vi "EnvironmentStepAnanlysisModule.vi"(0 "AnalysisContext":refnum<k7>) -> (1 "status":bool, 2 "code":i32, 3 "source":string)   [LabVIEW 2013]
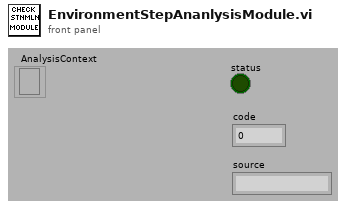
[diagram p1: front panel]
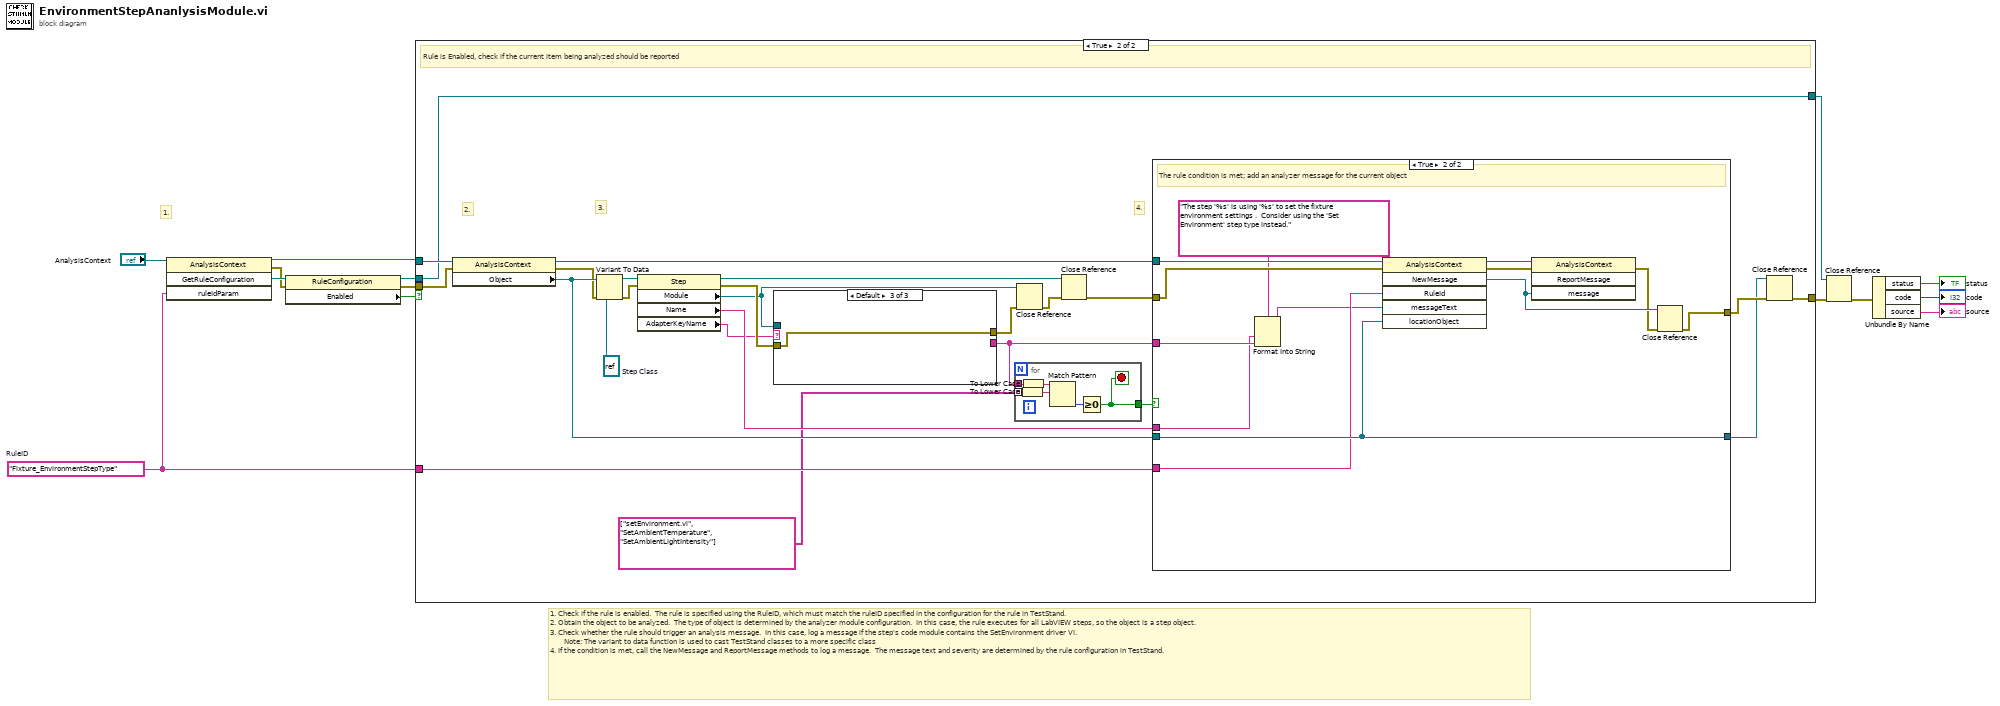
[diagram p0: block diagram]
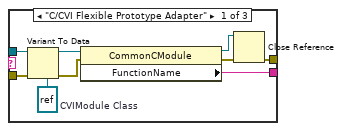
[diagram p3: hidden frame]
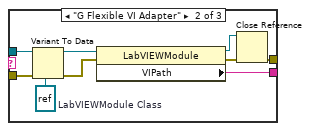
[diagram p4: hidden frame]
diagram:
  w6 = "Fixture_EnvironmentStepType"  # RuleID
  # "1. Check if the rule is enabled.  The rule is specified using the RuleID, which must match the ruleID specified in the configuration for the rule in TestStand.\n2. Obtain the object to be analyzed.  The type of object is determined by the analyzer module configuration.  In this case, the rule executes for all LabVIEW steps, so the object is a step object.\n3. Check whether the rule should trigger an analysis message.  In this case, log a message if the step's code module contains the SetEnvironment driver VI.  \n       Note: The variant to data function is used to cast TestStand classes to a more specific class\n4. If the condition is met, call the NewMessage and ReportMessage methods to log a message.  The message text and severity are determined by the rule configuration in TestStand."
  # "1."
  n1 = invoke class="AnalysisContext" method="GetRuleConfiguration"(reference="AnalysisContext", "ruleIdParam"=w6) -> (reference out=w10:refnum<k7>, error out=w12:errorcluster, "GetRuleConfiguration"=w13:refnum<k7>)  [unwired: 2 in, 1 out]
  n2 = property class="RuleConfiguration"(reference=w13, error in=w12) -> (reference out=w5:refnum<k7>, error out=w4:errorcluster, "Enabled"=w11:bool)
  n3 = case shown="True" w11 {
    tunnel: w4 -> [w16 w19]
    tunnel: [w16 w27] -> w3
    tunnel: w10 -> [_ w23]
    tunnel: w6 -> [_ w25]
    tunnel: w5 -> [w15 w20]
    tunnel: [w15 w20] -> w2
    frame False {
      # "Rule is Disabled, do nothing"
    }
    frame True {
      w39 = refnum<k7> refnum  # Step Class
      # "4."
      # "3."
      # "2."
      # "Rule is Enabled, check if the current item being analyzed should be reported"
      n4 = property class="AnalysisContext"(reference=w23, error in=w19) -> (reference out=w40:refnum<k7>, error out=w18:errorcluster, "Object"=w29:refnum<k7>)
      n5 = Variant To Data(error in=w18, type=w39, Variant=w29) -> (data=w38:refnum<k7>, error out=w37:errorcluster)
      n6 = property class="Step"(reference=w38, error in=w37) -> (reference out=w31:refnum<k7>, error out=w36:errorcluster, "Module"=w33:refnum<k7>, "Name"=w24:string, "AdapterKeyName"=w17:string)
      n7 = case shown="Default" w17 {
        tunnel: w36 -> [w47 w62 w65]
        tunnel: [w49 w58 w65] -> w34
        tunnel: w33 -> [w52 w57 _]
        tunnel: [w50 w56 _] -> w22
        frame "C/CVI Flexible Prototype Adapter" {
          w51 = refnum<k7> refnum  # CVIModule Class
          n8 = Variant To Data(error in=w47, type=w51, Variant=w52) -> (data=w55:refnum<k7>, error out=w54:errorcluster)
          n9 = property class="CommonCModule"(reference=w55, error in=w54) -> (reference out=w48:refnum<k7>, error out=w53:errorcluster, "FunctionName"=w50:string)
          n10 = Close Reference(reference=w48, error in (no error)=w53) -> (error out=w49:errorcluster)
        }
        frame "G Flexible VI Adapter" {
          w64 = refnum<k7> refnum  # LabVIEWModule Class
          n11 = Variant To Data(error in=w62, type=w64, Variant=w57) -> (data=w63:refnum<k7>, error out=w61:errorcluster)
          n12 = property class="LabVIEWModule"(reference=w63, error in=w61) -> (reference out=w60:refnum<k7>, error out=w59:errorcluster, "VIPath"=w56:string)
          n13 = Close Reference(reference=w60, error in (no error)=w59) -> (error out=w58:errorcluster)
        }
        frame Default {
        }
      }
      n14 = for {
        tunnel: [w41] -> w35
        tunnel: w22 -> [w43]
        tunnel: string[] ["setEnvironment.vi", "SetAmbientTemperature", "SetAmbientLightIntensity"] -> [w42] mode=indexing
        stop <- w41 stop-if-true
        n15 = To Lower Case(string=w42) -> (all lower case string=w45:string)
        n16 = To Lower Case(string=w43) -> (all lower case string=w44:string)
        n17 = Match Pattern(string=w44, regular expression=w45) -> (offset past match=w46:i32)  [unwired: 1 in, 3 out]
        n18 = Greater Or Equal To 0?(x=w46) -> (x >= 0?=w41:bool)
      }
      n19 = Close Reference(reference=w33, error in (no error)=w34) -> (error out=w32:errorcluster)
      n20 = Close Reference(reference=w31, error in (no error)=w32) -> (error out=w30:errorcluster)
      n21 = case shown="True" w35 {
        tunnel: [w67 w80] -> w28
        tunnel: w40 -> [_ w75]
        tunnel: w30 -> [w67 w76]
        tunnel: w29 -> [w66 w73]
        tunnel: [w66 w73] -> w26
        tunnel: w25 -> [_ w72]
        tunnel: w22 -> [_ w71]
        tunnel: w24 -> [_ w68]
        frame False {
          # "Condition was not met, do nothing"
        }
        frame True {
          # "The rule condition is met; add an analyzer message for the current object"
          n22 = Format Into String(format string="The step '%s' is using '%s' to set the fixture environment settings .  Consider using the 'Set Environment' step type instead." ("messageText"), w68, w71) -> (resulting string=w69:string)  [unwired: 2 in, 1 out]
          n23 = invoke class="AnalysisContext" method="NewMessage"(reference=w75, error in=w76, "RuleId"=w72, "messageText"=w69, "locationObject"=w73) -> (reference out=w79:refnum<k7>, error out=w78:errorcluster, "NewMessage"=w77:refnum<k7>)  [unwired: 1 in, 3 out]
          n24 = invoke class="AnalysisContext" method="ReportMessage"(reference=w79, error in=w78, "message"=w77) -> (error out=w74:errorcluster)  [unwired: 1 in, 3 out]
          n25 = Close Reference(reference=w77, error in (no error)=w74) -> (error out=w80:errorcluster)
        }
      }
      n26 = Close Reference(reference=w26, error in (no error)=w28) -> (error out=w27:errorcluster)
    }
  }
  n27 = Close Reference(reference=w2, error in (no error)=w3) -> (error out=w1:errorcluster)
  n28 = Unbundle By Name(w1) -> ("status"=→"status":bool, "code"=→"code":i32, "source"=→"source":string)
